vi "9.2.vi"() -> ()   [LabVIEW 2017]
panel:
  out "sum":i32
  in  "String":string
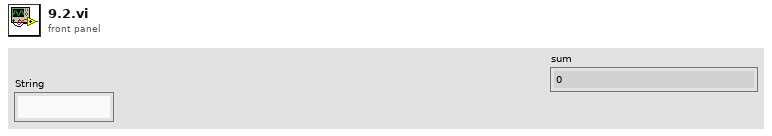
[diagram p1: front panel]
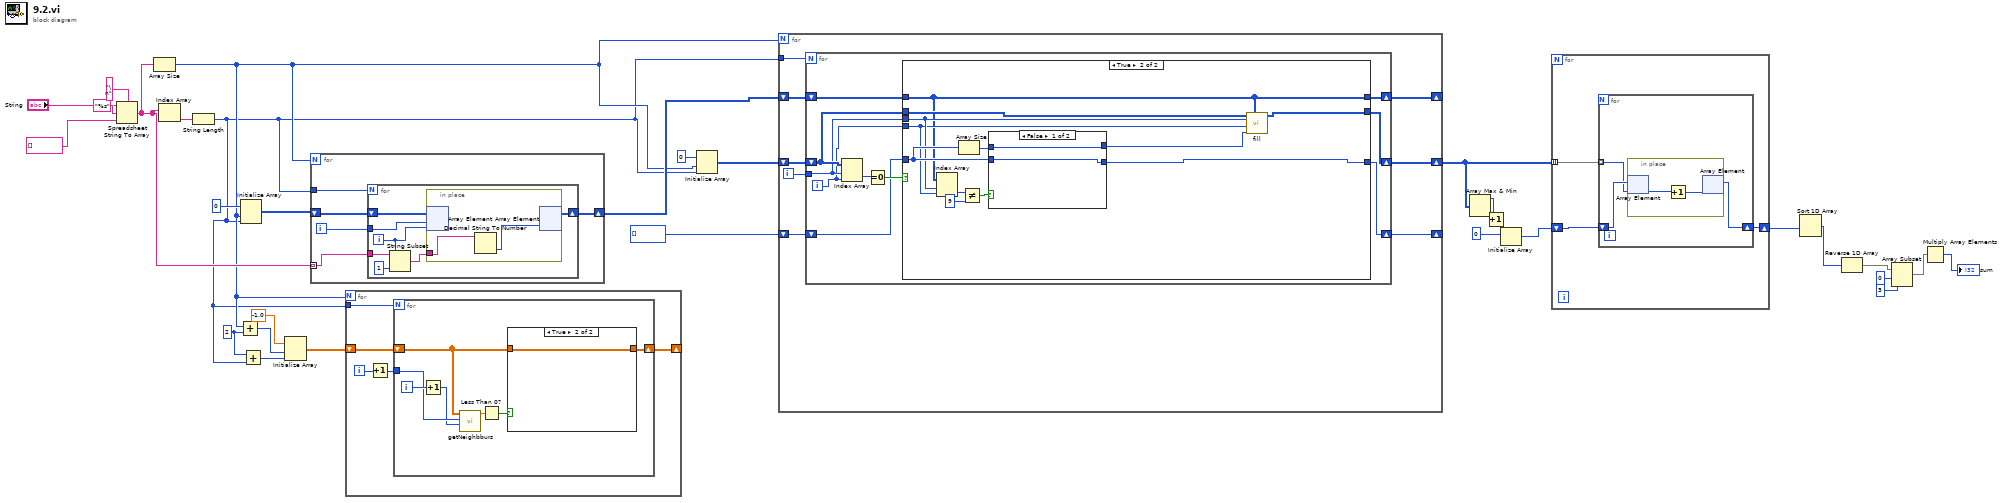
[diagram p0: block diagram]
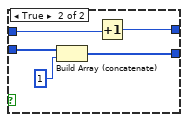
[diagram p4: hidden frame]
diagram:
  w19 = 2 ("y")
  n1 = Spreadsheet String To Array(delimiter (Tab)="\n", format string="%s", spreadsheet string="String", array type (2D Dbl)=string[] []) -> (array=w22:string[])
  n2 = Array Size(array=w22) -> (size(s)=w14:i32)
  n3 = Index Array(array=w22) -> (element=w27:string)  [unwired: 1 in]
  n4 = String Length(string=w27) -> (length=w13:i32)
  n5 = Add(x=w14, y=w19) -> (x+y=w18:i32)
  n6 = Initialize Array(0, w14, w13) -> (w23:i32[][])
  n7 = Add(x=w19, y=w13) -> (x+y=w17:i32)
  n8 = Initialize Array(-1.0 ("element"), w18, w17) -> (w15:dbl[][])
  n9 = for {
    N: w14 -> [_]
    tunnel: w13 -> [w36]
    shift-right: [w34] -> w21
    shift-left: w23 -> [w35]
    tunnel: w22 -> [w32] mode=indexing
    i -> [w33]
    n10 = for {
      N: w36 -> [_]
      shift-right: [w38] -> w34
      shift-left: w35 -> [w43]
      tunnel: w33 -> [w42]
      tunnel: w32 -> [w40]
      i -> [w37]
      n11 = String Subset(string=w40, offset (0)=w37, length (rest)=1 ("length (rest)")) -> (substring=w39:string)
      n12 = in-place {
        in-place-border: w39 -> [w45]
        n13 = in-place-array #1(w43, w42, w37) -> ()  [unwired: 1 out]
        n14 = Decimal String To Number(string=w45) -> (number=w44:i32)  [unwired: 2 in, 1 out]
        n15 = in-place-array #1(w44) -> (w38:i32[][])  [unwired: 2 out]
      }
    }
  }
  n16 = for {
    N: w14 -> [_]
    tunnel: w13 -> [w50]
    shift-right: [w46] -> _
    shift-left: w15 -> [w49]
    i -> [w48]
    n17 = Increment(x=w48) -> (x+1=w47:i32)
    n18 = for {
      N: w50 -> [_]
      tunnel: w47 -> [w56]
      shift-right: [w51] -> w46
      shift-left: w49 -> [w52]
      i -> [w57]
      n19 = Increment(x=w57) -> (x+1=w55:i32)
      n20 = call "getNeighbburs.vi"("col"=w55, "row"=w56, "Array"=w52) -> ("element"=w54:dbl)  [unwired: 7 in, 1 out]
      n21 = Less Than 0?(x=w54) -> (x < 0?=w53:bool)
      n22 = case shown="True" w53 {
        tunnel: w52 -> [w58 w59]
        tunnel: [w58 w59] -> w51
        frame False {
        }
        frame True {
        }
      }
    }
  }
  n23 = Initialize Array(0, w14, w13) -> (w26:i32[][])
  n24 = for {
    N: w14 -> [_]
    tunnel: w13 -> [w67]
    shift-right: [w63] -> _
    shift-left: w21 -> [w64]
    shift-right: [w62] -> w12
    shift-left: w26 -> [w66]
    shift-right: [w60] -> _
    shift-left: i32[] [] -> [w61]
    i -> [w65]
    n25 = for {
      N: w67 -> [_]
      tunnel: w65 -> [w69]
      shift-right: [w73] -> w63
      shift-left: w64 -> [w74]
      shift-right: [w72] -> w62
      shift-left: w66 -> [w75]
      shift-right: [w71] -> w60
      shift-left: w61 -> [w70]
      i -> [w68]
      n26 = Index Array(array=w75, index (row)=w69, index (col)=w68) -> (element=w77:i32)
      n27 = Equal To 0?(x=w77) -> (x = 0?=w76:bool)
      n28 = case shown="True" w76 {
        tunnel: w75 -> [w79 w88]
        tunnel: w74 -> [w80 w81]
        tunnel: [w80 w81] -> w73
        tunnel: [w79 w90] -> w72
        tunnel: [w78 w91] -> w71
        tunnel: w70 -> [w78 w92]
        tunnel: w69 -> [_ w87]
        tunnel: w68 -> [_ w86]
        frame False {
        }
        frame True {
          n29 = Index Array(array=w81, index (row)=w87, index (col)=w86) -> (element=w85:i32)
          n30 = Array Size(array=w92) -> (size(s)=w82:i32)
          n31 = Not Equal?(x=w85, y=9) -> (x != y?=w83:bool)
          n32 = case shown="False" w83 {
            tunnel: w92 -> [w93 w99]
            tunnel: [w93 w98] -> w91
            tunnel: [w94 w96] -> w89
            tunnel: w82 -> [w94 w95]
            frame False {
            }
            frame True {
              n33 = Build Array (concatenate)(w99, 1) -> (w98:i32[])
              n34 = Increment(x=w95) -> (x+1=w96:i32)
            }
          }
          n35 = call "fill.vi"("depth"=w81, "index"=w89, "col"=w86, "row"=w87, "basins"=w88) -> ("basins out"=w90:i32[][])  [unwired: 6 in]
        }
      }
    }
  }
  n36 = Array Max & Min(array=w12) -> (max value=w11:i32)  [unwired: 3 out]
  n37 = Increment(x=w11) -> (x+1=w8:i32)
  n38 = Initialize Array(0, w8) -> (w9:i32[])
  n39 = for {
    tunnel: w12 -> [w102] mode=indexing
    shift-right: [w100] -> w7
    shift-left: w9 -> [w101]
    n40 = for {
      tunnel: w102 -> [w104] mode=indexing
      shift-right: [w103] -> w100
      shift-left: w101 -> [w105]
      n41 = in-place {
        n42 = in-place-array #2(w105, w104) -> (w107:i32)
        n43 = Increment(x=w107) -> (x+1=w106:i32)
        n44 = in-place-array #2(w106) -> (w103:i32[])  [unwired: 1 out]
      }
    }
  }
  n45 = Sort 1D Array(array=w7) -> (sorted array=w6:i32[])
  n46 = Reverse 1D Array(array=w6) -> (reversed array=w5:i32[])
  n47 = Array Subset(array=w5, index=0, length=3) -> (w2:i32[])
  n48 = Multiply Array Elements(1:w2) -> (0:→"sum":i32)
